vi "Init_var.vi"() -> ()   [LabVIEW 2019]
panel:
  in  "Init":bool
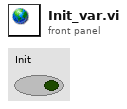
[diagram p1: front panel]
diagram:
